vi "Final-MurphyE-MultiFindCOM.vi"(0 "Name of Desired\nInstrument":string="E3631A") -> (1 "Number of Active\nCOM Ports":i32, 2 "List of Active Com Ports":refnum<visa-resource-name>[](array[refnum]), 3 "Desired COM Port Array":refnum<visa-resource-name>[](array[refnum]), 4 "Instrument (s)\nNot Found":bool)   [LabVIEW 2019]
doc: "Searches all the active COM ports for an instrument that responds to a *idn? query with a response that includes the text given as \"Name of Desired Instrument\".\nThe list of active COM ports includes instruments that don't even respond to such queries."
uses:
  <vilib>/Instr/_visa.llb/VISA Configure Serial Port (Instr).vi
panel:
  out "Instrument Responses":string[](array[string])
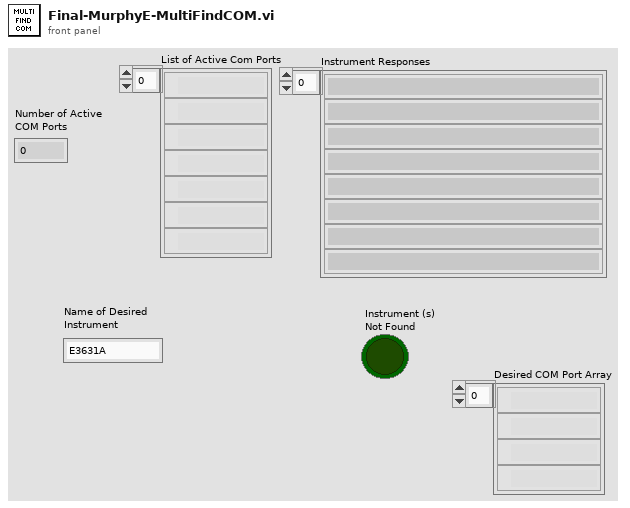
[diagram p1: front panel]
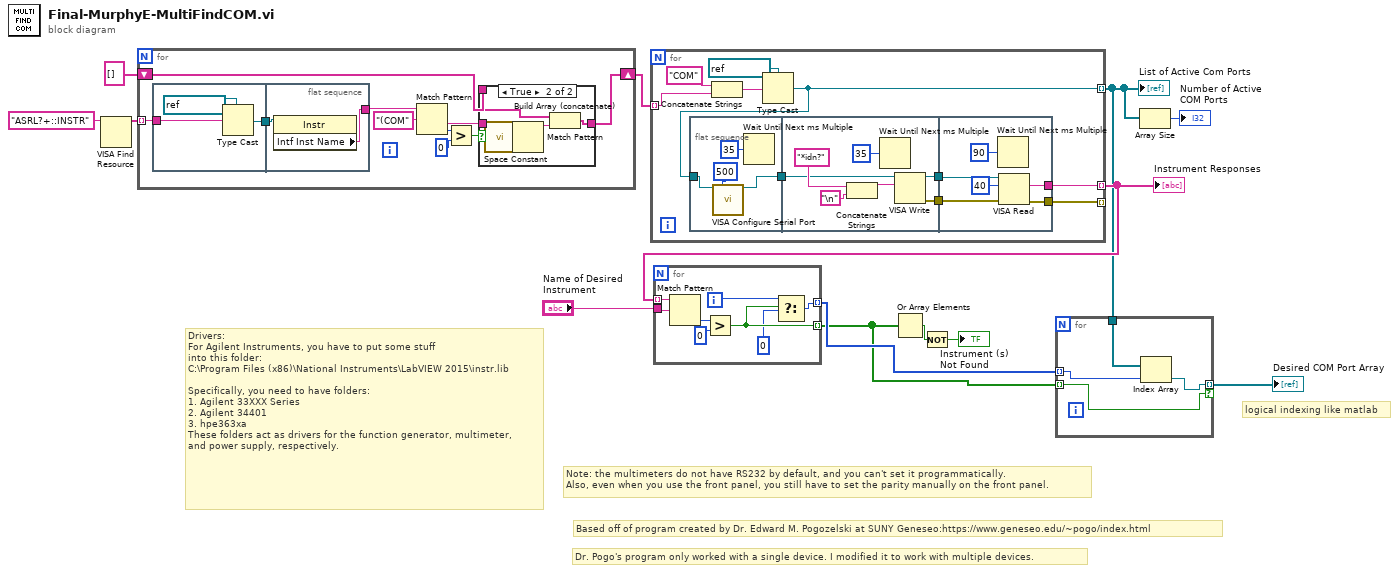
[diagram p0: block diagram]
diagram:
  # "Dr. Pogo's program only worked with a single device. I modified it to work with multiple devices."
  # "Based off of program created by Dr. Edward M. Pogozelski at SUNY Geneseo:https://www.geneseo.edu/~pogo/index.html"
  # "logical indexing like matlab"
  # "Drivers:\nFor Agilent Instruments, you have to put some stuff\ninto this folder:\nC:\\Program Files (x86)\\National Instruments\\LabVIEW 2015\\instr.lib\n\nSpecifically, you need to have folders:\n1. Agilent 33XXX Series \n2. Agilent 34401 \n3. hpe363xa\nThese folders act as drivers for the function generator, multimeter,\nand power supply, respectively."
  # "Note: the multimeters do not have RS232 by default, and you can't set it programmatically.\nAlso, even when you use the front panel, you still have to set the parity manually on the front panel."
  n1 = VISA Find Resource(11:"ASRL?+::INSTR" ("expression (\"?*\")")) -> (3:w12:string[])  [unwired: 2 in, 2 out]
  n2 = for {
    tunnel: w12 -> [w23] mode=indexing
    shift-right: [w14] -> w10
    shift-left: string[] [] -> [w15]
    n3 = flat-sequence {
      tunnel: w23 -> [w31]
      tunnel: [w30] -> w22
      tunnel: w22 -> [w34]
      tunnel: [w33] -> w21
      frame #0 {
        n4 = Type Cast(type=refnum<visa-resource-name> "COM1" ("Com Port?"), x=w31) -> (*(type *) &x=w30:refnum<visa-resource-name>)
      }
      frame #1 {
        n5 = property class="Instr"(reference=w34) -> ("Intf Inst Name"=w33:string)  [unwired: 1 in, 2 out]
      }
    }
    n6 = Match Pattern(string=w21, regular expression="(COM") -> (after substring=w16:string, offset past match=w19:i32)  [unwired: 1 in, 2 out]
    n7 = Greater?(x=w19, y=0) -> (0:w17:bool)
    n8 = case shown="True" w17 {
      tunnel: w16 -> [_ w29]
      tunnel: w15 -> [w24 w26]
      tunnel: [w24 w25] -> w14
      frame False {
      }
      frame True {
        n9 = call <vilib>:"Space Constant.vi"() -> ("String"=w28:string)
        n10 = Match Pattern(string=w29, regular expression=w28) -> (before substring=w27:string)  [unwired: 1 in, 3 out]
        n11 = Build Array (concatenate)(w26, w27) -> (w25:string[])
      }
    }
  }
  n12 = for {
    tunnel: w10 -> [w41] mode=indexing
    tunnel: [w35] -> w3 mode=indexing
    tunnel: [w39] -> w5 mode=indexing
    tunnel: [w38] -> _ mode=indexing
    n13 = flat-sequence {
      tunnel: w35 -> [w47]
      tunnel: [w46] -> w36
      tunnel: [w50] -> w40
      tunnel: [w49] -> w37
      tunnel: w36 -> [w51]
      tunnel: w40 -> [w59]
      tunnel: [w58] -> w39
      tunnel: [w57] -> w38
      tunnel: w37 -> [w56]
      frame #0 {
        n14 = call-poly "VISA Configure Serial Port"("VISA resource name"=w47, "timeout (10sec)"=u32 500) -> ("VISA resource name out"=w46:refnum<visa-resource-name>)  [unwired: 12 in, 1 out]
        n15 = Wait Until Next ms Multiple(millisecond multiple=u32 35) -> ()  [unwired: 1 out]
      }
      frame #1 {
        n16 = Concatenate Strings("*idn?", "\n") -> (w54:string)
        n17 = Wait Until Next ms Multiple(millisecond multiple=u32 35) -> ()  [unwired: 1 out]
        n18 = VISA Write(VISA resource name=w51, write buffer=w54) -> (VISA resource name out=w50:refnum<visa-resource-name>, error out=w49:errorcluster)  [unwired: 1 in, 1 out]
      }
      frame #2 {
        n19 = Wait Until Next ms Multiple(millisecond multiple=u32 90) -> ()  [unwired: 1 out]
        n20 = VISA Read(VISA resource name=w59, byte count=u32 40, error in (no error)=w56) -> (read buffer=w58:string, error out=w57:errorcluster)  [unwired: 2 out]
      }
    }
    n21 = Concatenate Strings("COM" ("string"), w41) -> (w42:string)
    n22 = Type Cast(type=refnum<visa-resource-name> "COM1" ("Com Port?"), x=w42) -> (*(type *) &x=w35:refnum<visa-resource-name>)
  }
  "List of Active Com Ports" <- w3
  "Instrument Responses" <- w5
  n23 = for {
    tunnel: w5 -> [w68] mode=indexing
    tunnel: "Name of Desired\nInstrument" -> [w69]
    tunnel: [w65] -> w1 mode=indexing
    tunnel: [w63] -> w4 mode=indexing
    i -> [w62]
    n24 = Match Pattern(string=w68, regular expression=w69) -> (offset past match=w67:i32)  [unwired: 1 in, 3 out]
    n25 = Greater?(x=w67, y=0) -> (0:w65:bool)
    n26 = Select(t=w62, s=w65, f=0) -> (s? t:f=w63:i32)
  }
  n27 = Or Array Elements(Boolean array=w1) -> (logical OR=w7:bool)
  n28 = Not(x=w7) -> (.not. x?=→"Instrument (s)\nNot Found":bool)
  n29 = for {
    tunnel: w4 -> [w72] mode=indexing
    tunnel: w3 -> [w73]
    tunnel: [w71] -> w2 mode=indexing if=w70
    tunnel: w1 -> [w70] mode=indexing
    n30 = Index Array(array=w73, index=w72) -> (element=w71:refnum<visa-resource-name>)
  }
  "Desired COM Port Array" <- w2
  n31 = Array Size(array=w3) -> (size(s)=→"Number of Active\nCOM Ports":i32)
